vi "Set Symmetry Analog Out.vi"(7 "percentageSymmetry":dbl=50.0, 8 "error in (no error)":errorcluster, 9 "node":T1, 10 "idxChannel":i32, 11 "hdwf":i32) -> (0 "error out":errorcluster, 3 "hdwf out":i32)   [LabVIEW 2014, in "AnalogDiscSDKLv.lvlib"]
doc: "extern \"C\" __declspec(dllexport) int SetSymmetry_AnalogOut(\n HDWF hdwf,\n int idxChannel,\n AnalogOutNode node,\n double percentageSymmetry );"
uses:
  <instrlib>/AnalogDiscSDKLv/AnalogDiscSDKLv.lvlib
  <instrlib>/AnalogDiscSDKLv/VIs/DWF_Node.ctl
  <instrlib>/AnalogDiscSDKLv/AnalogDiscSDKLv.dll
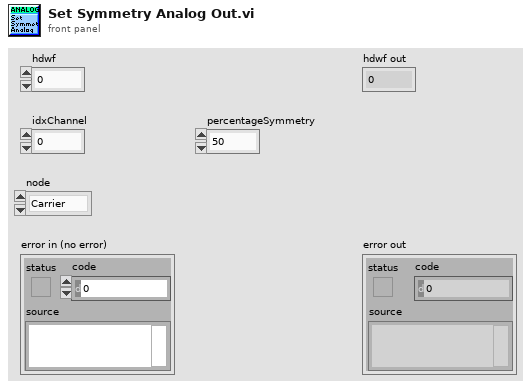
[diagram p1: front panel]
types:
  T1 = typedef "AnalogDiscSDKLv.lvlib/DWF_Node.ctl" = enum16{"Carrier", "FM", "AM"}
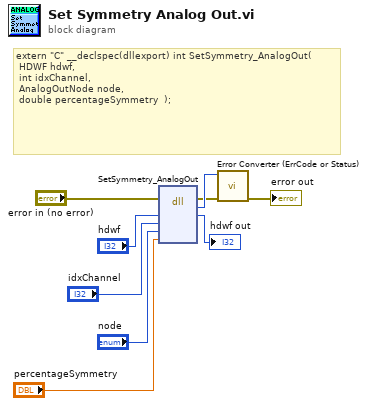
[diagram p0: block diagram]
diagram:
  # "extern \"C\" __declspec(dllexport) int SetSymmetry_AnalogOut(\n\tHDWF hdwf,\n\tint idxChannel,\n\tAnalogOutNode node,\n\tdouble percentageSymmetry\t\t);"
  n1 = dll-call lib="C:/Program Files (x86)/National Instruments/LabVIEW 2014/instr.lib/AnalogDiscSDKLv/AnalogDiscSDKLv.*" fn="SetSymmetry_AnalogOut"(error in="error in (no error)", "hdwf"="hdwf", "idxChannel"="idxChannel", "node"="node", "percentageSymmetry"="percentageSymmetry") -> (error out=w2:errorcluster, w3:i32, "hdwf"=→"hdwf out":i32)  [unwired: 5 in, 1 out]
  n2 = call <instrlib>:"Error Converter (ErrCode or Status).vi"("error in (no error)"=w2, "error code"=w3) -> ("error out"=→"error out":errorcluster)  [unwired: 9 in]
